vi "LVClass_SlopesPostProcessList ctor from has.vi"(0 "SlopesPostProcessorList in":refnum<class "SlopesPostProcessorList.lvclass">, 5 "has file path":path, 11 "error in (no error)":errorcluster) -> (4 "SlopesPostProcessorList out":refnum<class "SlopesPostProcessorList.lvclass">, 15 "error out":errorcluster)   [LabVIEW 2020, in "SlopesPostProcessorList.lvclass"]
doc: "SlopesPostProcessorList constructor from a .has file.\n\n--------------------------------------------------------------------------------\n\n<B>SlopesPostProcessorIn </B> : Constant Pointer to SlopesPostProcessorList object.\n<B>SlopesPostProcessorOut </B> : Constant Pointer to SlopesPostProcessorList object.\n<B>HAS_FilePath </B> : Path to .has file.\n<B>ErrorIn </B> : Error\n<B>ErrorOut </B> : Error\n\n--------------------------------------------------------------------------------"
uses:
  SlopesPostProcessorList.lvclass
  Handle creation.ctl
  SlopesPostProcessorList.lvclass/SlopesPostProcessorList.ctl
  HasoSlopes.lvclass
  Pupil.lvclass
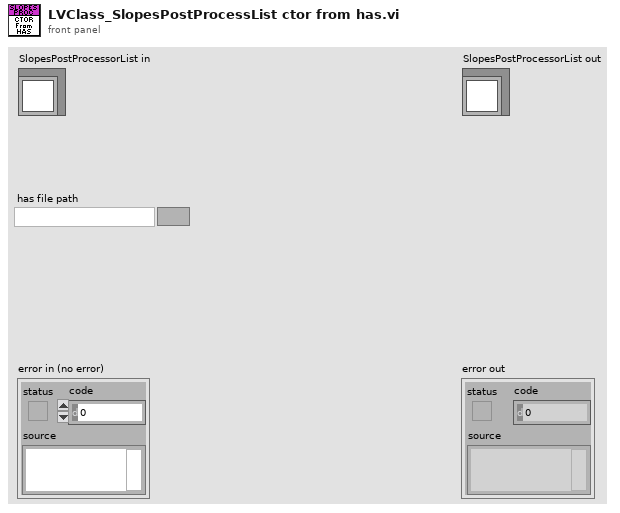
[diagram p1: front panel]
types:
  T1 = typedef "Handle creation.ctl" = enum16{"By ctor", "By write function"}
  T2 = typedef "HAS File information.ctl" = cluster{"SerialNumber":string, "HasoModel":string, "Revision":u32, "Dimension_um":T3, "Lower calibration wavelength (nm)":dbl, "Upper calibration wavelength (nm)":dbl, "Acquistion time":timestamp, "Source wavelength (nm)":dbl, "Session name":string, "Comment":string, "FileVersion":i32}
  T3 = typedef "General dimensions definition.ctl" = cluster{"Size":T4, "Step":T5}
  T4 = typedef "Point2D.ctl" = cluster{"X":u32, "Y":u32}
  T5 = typedef "Point2Df.ctl" = cluster{"X":sgl, "Y":sgl}
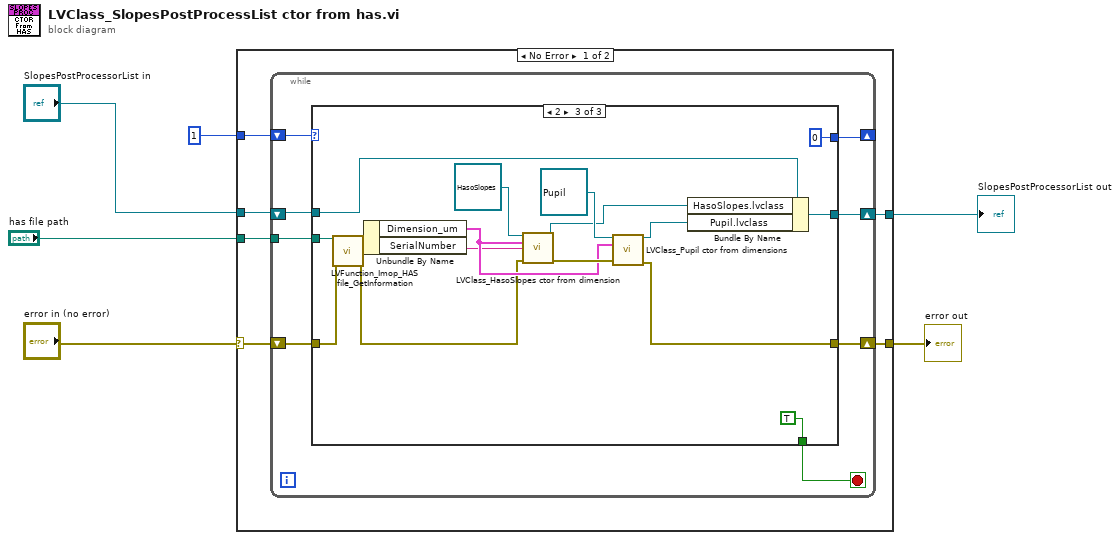
[diagram p0: block diagram]
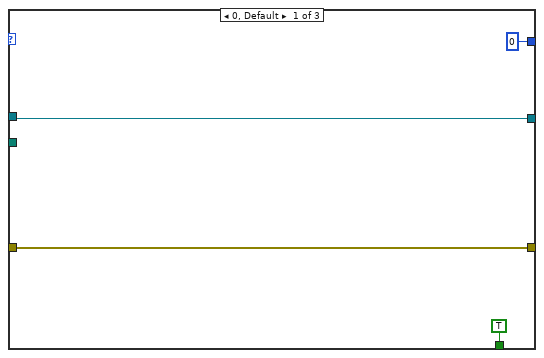
[diagram p2: hidden frame]
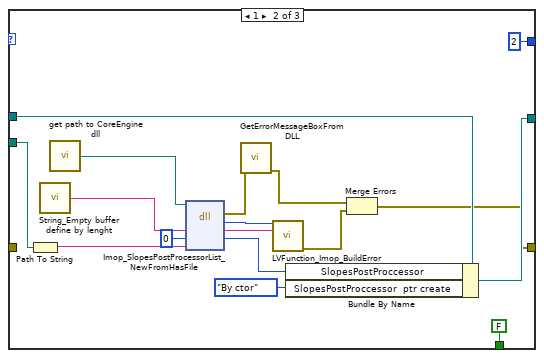
[diagram p3: hidden frame]
diagram:
  n1 = case shown="No Error" "error in (no error)" {
    selector: "error in (no error)" -> [w8 w58]
    tunnel: "SlopesPostProcessorList in" -> [w10 w59]
    tunnel: [w12 w59] -> w3
    tunnel: [w11 w58] -> w2
    tunnel: 1 -> [w9 _]
    tunnel: "has file path" -> [w7 _]
    frame No Error {
      n2 = while {
        shift-right: [w16] -> _
        shift-left: w9 -> [w17]
        shift-right: [w19] -> w11
        shift-left: w8 -> [w15]
        shift-right: [w20] -> w12
        shift-left: w10 -> [w18]
        tunnel: w7 -> [w13]
        stop <- w14 stop-if-true
        n3 = case shown="2" w17 {
          tunnel: [w22 w41 w50] -> w20
          tunnel: [w23 w34 w54] -> w19
          tunnel: w18 -> [w22 w40 w53]
          tunnel: [0 2 0] -> w16
          tunnel: w15 -> [w23 _ w43]
          tunnel: [TRUE FALSE TRUE] -> w14
          tunnel: w13 -> [_ w26 w47]
          frame 0, Default {
          }
          frame 1 {
            n4 = Path To String(path=w26) -> (string=w25:string)
            n5 = call "String_Empty buffer define by lenght.vi"() -> ("Empty buffer"=w33:string)  [unwired: 1 in]
            n6 = call "get path to CoreEngine dll.vi"() -> ("path to c_interface_vc100.dll"=w32:path)  [unwired: 12 in, 3 out]
            n7 = dll-call lib="D:/soft/HASO_v3/SVN_trunk/ImOpCoreEngine4_LV2011/DLLs/c_interface_vc100.dll" fn="Imop_SlopesPostProcessorList_NewFromHasFile"(path in=w32, "message"=w33, "objet"=0, "Has path"=w25) -> (error out=w27:errorcluster, "return type"=w29:i32, "message"=w28:string, "objet"=w30:i32)  [unwired: 3 in, 1 out]
            n8 = call "GetErrorMessageBoxFromDLL.vi"("error IN"=w27) -> ("error OUT"=w36:errorcluster)  [unwired: 10 in]
            n9 = call "LVFunction_Imop_BuildError.vi"("code"=w29, "String to Prepend to source (\"\")"=w28) -> ("error out"=w35:errorcluster)  [unwired: 13 in]
            n10 = Bundle By Name(cluster=w40, "SlopesPostProccessor"=w30, "SlopesPostProccessor  ptr create"=Handle_creation."By ctor" ("Slopes PP  ptr create")) -> (w41:refnum<class "SlopesPostProcessorList.lvclass">)
            n11 = Merge Errors(w36, w35) -> (w34:errorcluster)
          }
          frame 2 {
            n12 = call "LVFunction_Imop_HAS file_GetInformation.vi"("HAS file path"=w47, "error in (no error)"=w43) -> ("HAS file information"=w46:T2, "error out"=w42:errorcluster)  [unwired: 12 in]
            n13 = Unbundle By Name(w46) -> ("Dimension_um"=w45:T3, "SerialNumber"=w44:string)
            n14 = call "LVClass_HasoSlopes ctor from dimension.vi"("HasoSlopes in"=refnum<class "HasoSlopes.lvclass"> refnum, "Dimensions_um"=w45, "serial"=w44, "error in (no error)"=w42) -> ("HasoSlopes out"=w52:refnum<class "HasoSlopes.lvclass">, "error out"=w56:errorcluster)  [unwired: 10 in]
            n15 = call "LVClass_Pupil ctor from dimensions.vi"("Pupil in"=refnum<class "Pupil.lvclass"> refnum, "Dimensions_um"=w45, "error in (no error)"=w56) -> ("Pupil out"=w51:refnum<class "Pupil.lvclass">, "error out"=w54:errorcluster)  [unwired: 11 in]
            n16 = Bundle By Name(cluster=w53, "HasoSlopes.lvclass"=w52, "Pupil.lvclass"=w51) -> (w50:refnum<class "SlopesPostProcessorList.lvclass">)
          }
        }
      }
    }
    frame Error {
    }
  }
  "error out" <- w2
  "SlopesPostProcessorList out" <- w3
